vi "Configure Number of Envelopes.vi"(8 "error in (no error)":errorcluster {"code" format="%.0x"}, 10 "Number of Envelopes (16)":i32=16, 11 "VISA Resource Name":refnum<visa-resource-name>) -> (0 "error out":errorcluster {"code" format="%.0x"}, 3 "VISA Resource Name Out":refnum<visa-resource-name>)   [LabVIEW 2010, in "Tektronix TDS 3000 Series.lvlib"]
doc: "When you set the acquisition type to Envelope, the oscilloscope acquires multiple waveforms. After each waveform acquisition, the oscilloscope keeps the minimum and maximum values it finds for each element in the waveform record. This VI configures the number of waveforms the oscilloscope acquires and analyzes to create the minimum and maximum waveforms. \n\nAfter the oscilloscope acquires as many waveforms as specified, it returns to the idle state. \n\nNotes:\n\n(1) Set the Acquisition Type control to Envelope before you call this VI. To set the acquisition type, call the tktds3k Configure Acquisition Type VI."
uses:
  <instrlib>/Tektronix TDS 3000 Series/Tektronix TDS 3000 Series.lvlib
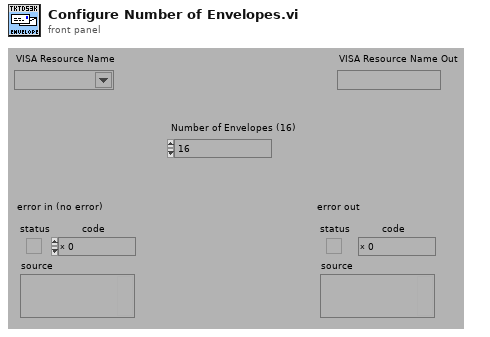
[diagram p1: front panel]
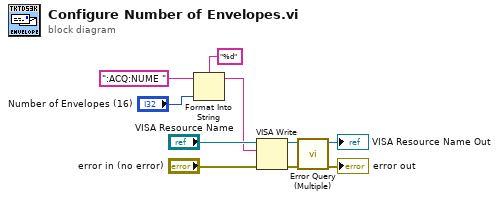
[diagram p0: block diagram]
diagram:
  n1 = Format Into String(format string="%d", initial string=":ACQ:NUME ", "Number of Envelopes (16)") -> (resulting string=w5:string)  [unwired: 1 in, 1 out]
  n2 = VISA Write(VISA resource name="VISA Resource Name", write buffer=w5, error in (no error)="error in (no error)") -> (VISA resource name out=w4:refnum<visa-resource-name>, error out=w3:errorcluster)  [unwired: 1 out]
  n3 = call <instrlib>:"Error Query (Multiple).vi"("error in (no error)"=w3, "VISA Resource Name"=w4) -> ("error out"=→"error out":errorcluster, "VISA Resource Name Out"=→"VISA Resource Name Out":refnum<visa-resource-name>)  [unwired: 6 in, 2 out]
